vi "proptest_instancecount.vi"() -> ()   [LabVIEW 2013, in "TBM Tests.lvlib"]
uses:
  TBM Tests.lvlib
  root configuration/TBM configuration.lvclass
panel:
  out "warning 538305":errorcluster
  out "no support=ok":bool
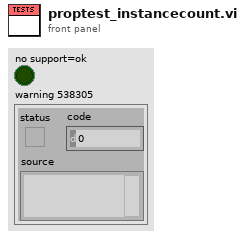
[diagram p1: front panel]
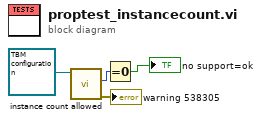
[diagram p0: block diagram]
diagram:
  n1 = call-dynamic "instance count allowed.vi"("configuration in"=refnum<class "TBM configuration.lvclass"> refnum ("configuration")) -> ("error out"=→"warning 538305":errorcluster, "instances allowed"=w2:i32)  [unwired: 8 in, 1 out]
  n2 = Equal To 0?(x=w2) -> (x = 0?=→"no support=ok":bool)
